vi "Wrapper for all VIs.vi"() -> ()   [LabVIEW 2017]
uses:
  examples/NEVSTOP/Communicable State Machine(CSM)/4. Advance Examples/6. Global Log Handling Capability/Global Log Handling Capability Example.lvlib
panel:
  in  "Name(\"\" to use uuid) 4":string="Event CSM Tiny"
  in  "Init State(\"Macro: Initialize\")":string="Macro: Initialize"
  in  "Name(\"\" to use uuid) 3":string="CSM-Module"
  in  "Name(\"\" to use uuid) 2":string="Event CSM"
  in  "Name(\"\" to use uuid)":string="Event CSM Tiny"
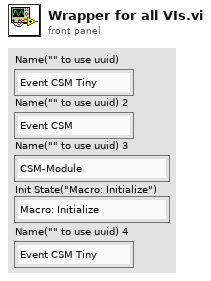
[diagram p1: front panel]
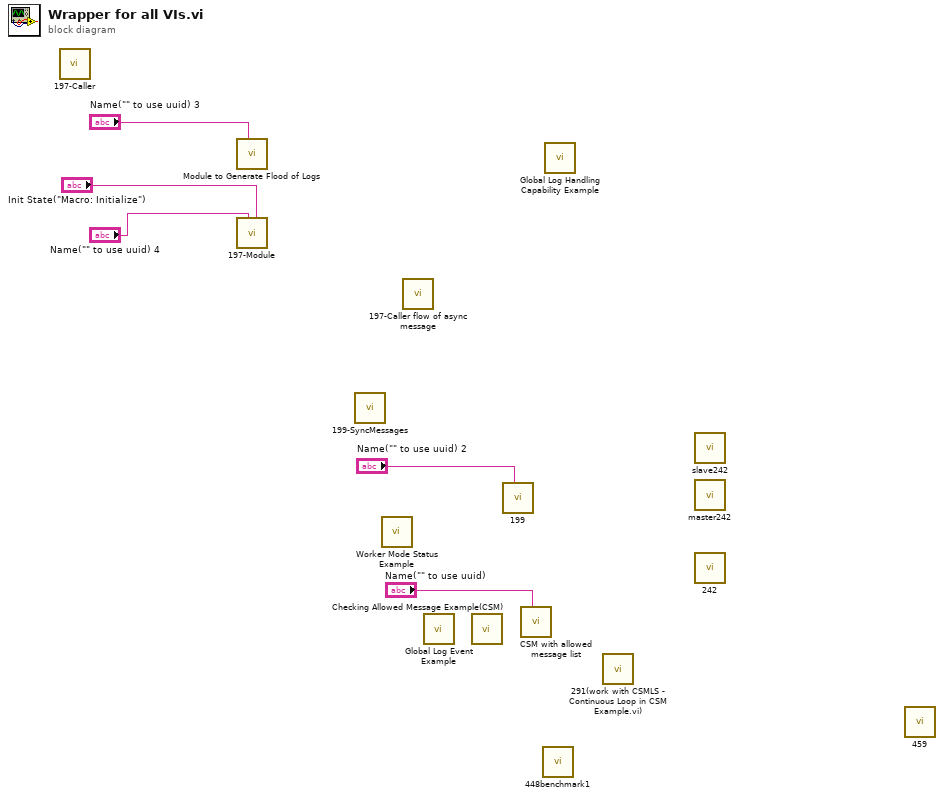
[diagram p0: block diagram]
diagram:
  n1 = call "197-Caller.vi"() -> ()  [unwired: 12 in]
  n2 = call "Module to Generate Flood of Logs.vi"("Name (\"\" to Use Uuid)"="Name(\"\" to use uuid) 3") -> ()  [unwired: 11 in]
  n3 = call "197-Module.vi"("Init State(\"Macro: Initialize\")"="Init State(\"Macro: Initialize\")", "Name(\"\" to use uuid)"="Name(\"\" to use uuid) 4") -> ()  [unwired: 10 in]
  n4 = call "199-SyncMessages.vi"() -> ()  [unwired: 12 in]
  n5 = call "Worker Mode Status Example.vi"() -> ()  [unwired: 12 in]
  n6 = call "197-Caller flow of async message.vi"() -> ()  [unwired: 12 in]
  n7 = call "Global Log Event Example.vi"() -> ()  [unwired: 12 in]
  n8 = call "Checking Allowed Message Example(CSM).vi"() -> ()  [unwired: 12 in]
  n9 = call "199.vi"("Name(\"\" to use uuid)"="Name(\"\" to use uuid) 2") -> ()  [unwired: 11 in]
  n10 = call "CSM with allowed message list.vi"("Name (\"\" to Use Uuid)"="Name(\"\" to use uuid)") -> ()  [unwired: 11 in]
  n11 = call "448benchmark1.vi"() -> ()  [unwired: 12 in]
  n12 = call "Global Log Handling Capability Example.vi"() -> ()  [unwired: 12 in]
  n13 = call "291(work with CSMLS - Continuous Loop in CSM Example.vi).vi"() -> ()  [unwired: 12 in]
  n14 = call "slave242.vi"() -> ()  [unwired: 12 in]
  n15 = call "master242.vi"() -> ()  [unwired: 12 in]
  n16 = call "242.vi"() -> ()  [unwired: 12 in]
  n17 = call "459.vi"() -> ()  [unwired: 12 in]
